vi "VisionGetDistanceToSpeakerGlobal.vi"() -> (3 "DistanceFromSpeaker(m)":dbl)   [LabVIEW 2023]
doc: "Gets the DistanceFromSpeaker Vision Global\nInputs: none\nOutputs: DistanceFromSpeaker--meters--numeric"
uses:
  VisionGlobal.vi
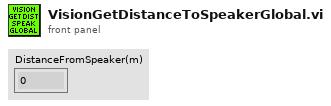
[diagram p1: front panel]
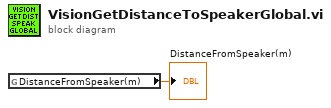
[diagram p0: block diagram]
diagram:
  n1 = global read "VisionGlobal.vi" "DistanceFromSpeaker(m)"() -> (→"DistanceFromSpeaker(m)":dbl)
